vi "Merge Error.vi"(10 "Error":errorcluster, 11 "Base Queue jettl in":refnum<class "Base Queue jettl.lvclass">) -> (3 "Base Queue jettl out":refnum<class "Base Queue jettl.lvclass">)   [LabVIEW 2021, in "jettl.lvlib" / "Base Queue jettl.lvlib" / "Base Queue jettl.lvclass"]
uses:
  Base Queue jettl.lvclass
  Base Queue jettl.lvclass/Base Queue jettl.ctl
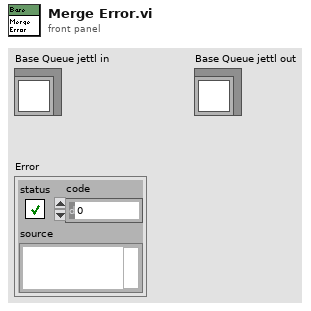
[diagram p1: front panel]
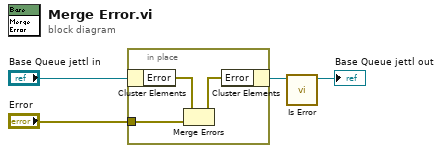
[diagram p0: block diagram]
diagram:
  n1 = in-place {
    in-place-border: "Error" -> [w5]
    n2 = in-place-cluster #1("Base Queue jettl in") -> ("Error"=w7:errorcluster)
    n3 = Merge Errors(w7, w5) -> (w6:errorcluster)
    n4 = in-place-cluster #1("Error"=w6) -> (w2:refnum<class "Base Queue jettl.lvclass">)
  }
  n5 = call "Is Error.vi"("Base Queue jettl in"=w2) -> ("Base Queue jettl out"=→"Base Queue jettl out":refnum<class "Base Queue jettl.lvclass">)  [unwired: 10 in]
